vi "CustomStartService.vi"(8 "error in":errorcluster, 11 "Server Address":string="localhost:50051") -> (0 "error out":errorcluster, 1 "Listening Port":i32, 2 "Server Stop":refnum<user-event>, 3 "gRPC Server out":refnum<class "Servicer.lvclass">, 5 "MicronUE":refnum<user-event>)   [LabVIEW 2019, in "MicronGRPCGeneratedServer.lvlib"]
uses:
  MicronGRPCGeneratedServer.lvlib
  <vilib>/gRPC/LabVIEW gRPC Servicer/Servicer/Servicer.lvclass
  Base/Server/Message/MessageBase.lvclass
  <vilib>/gRPC/LabVIEW gRPC Servicer/Servicer/Servicer.lvclass/Servicer.ctl
  RPC Service/MicronGRPC/MicronGRPC.lvclass
  C:/Program Files (x86)/National Instruments/LabVIEW 2019/vi.lib/gRPC/LabVIEW gRPC Servicer/ServiceBase/ServiceBase.lvclass
  SubVIs/CustomEventHandler.vi
panel:
  in  "Server Certificate File (.crt)":path
  in  "Server Key File (.key)":path
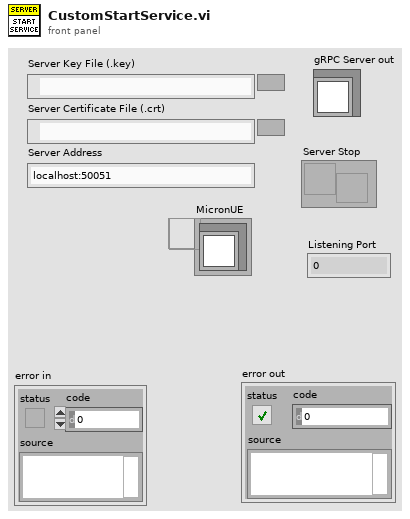
[diagram p1: front panel]
types:
  T1 = typedef "grpc-lvsupport-release.lvlib/grpcId.ctl" = u64
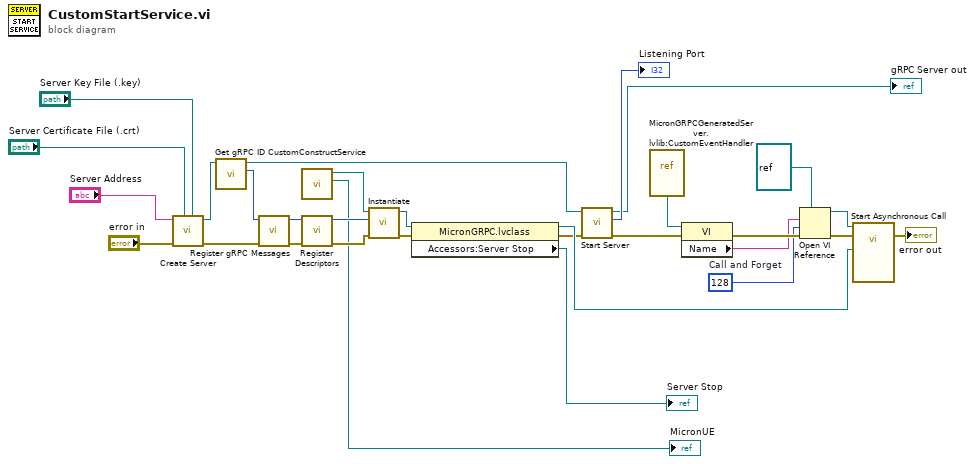
[diagram p0: block diagram]
diagram:
  w3 = 128  # Call and Forget
  n1 = call <vilib>:"Create Server.vi"("Server Key File (.key)"="Server Key File (.key)", "Server Certificate File (.crt)"="Server Certificate File (.crt)", "error in"="error in", "Server Address"="Server Address") -> ("error out"=w24:errorcluster, "gRPC Server out"=w26:refnum<class "Servicer.lvclass">)  [unwired: 6 in]
  n2 = call <vilib>:"Get gRPC ID.vi"("OOP Server in"=w26) -> ("gRPC ID"=w25:T1, "OOP Server out"=w21:refnum<class "Servicer.lvclass">)  [unwired: 9 in]
  n3 = call "Register gRPC Messages.vi"("error in (no error)"=w24, "gRPC ID"=w25) -> ("error out"=w23:errorcluster, "gRPC ID Out"=w22:T1)  [unwired: 8 in]
  n4 = call "CustomConstructService.vi"() -> ("MicronMessageUE"=→"MicronUE":refnum<user-event>, "MicronGRPC out"=w16:refnum<class "MicronGRPC.lvclass">)  [unwired: 10 in]
  n5 = call "Register Descriptors.vi"("error in (no error)"=w23, "gRPC ID"=w22) -> ("error out"=w20:errorcluster, "gRPC ID Out"=w19:T1)  [unwired: 8 in]
  n6 = call-dynamic "Instantiate.vi"("error in"=w20, "gRPCid"=w19, "iService"=w16) -> ("error out"=w17:errorcluster, "iService"=w18:refnum<class "MicronGRPC.lvclass">)  [unwired: 7 in]
  n7 = property class="MicronGRPC.lvclass"(reference=w18, error in=w17) -> (reference out=w15:refnum<class "MicronGRPC.lvclass">, error out=w14:errorcluster, "Accessors:Server Stop"=→"Server Stop":refnum<user-event>)
  n8 = call <vilib>:"Start Server.vi"("error in"=w14, "gRPC Server in"=w21) -> ("error out"=w4:errorcluster, "Listening Port"=→"Listening Port":i32, "gRPC Server out"=→"gRPC Server out":refnum<class "Servicer.lvclass">)  [unwired: 7 in]
  n9 = vi-ref "MicronGRPCGeneratedServer.lvlib:CustomEventHandler.vi"() -> (w2:refnum<vi>)
  n10 = property class="VI"(reference=w2, error in=w4) -> (error out=w7:errorcluster, "Name"=w6:string)  [unwired: 1 out]
  n11 = Open VI Reference(type specifier VI Refnum (for type only)=refnum<vi> refnum ("reference"), vi path=w6, options=w3, error in (no error)=w7) -> (vi reference=w8:refnum<vi>, error out=w9:errorcluster)  [unwired: 2 in]
  n12 = call-by-ref "Start Asynchronous Call"(reference=w8, error in=w9, "MicronGRPC.lvclass"=w15) -> (error out=→"error out":errorcluster)  [unwired: 11 in, 1 out]
